vi "SetBTI.vi"(8 "error in (no error)":errorcluster, 10 "bti_mode":u8) -> (0 "error out":errorcluster)   [LabVIEW 2015, in "ESLSCDLL.lvlib"]
uses:
  ESLSCDLL.lvlib
  Globals.vi
  ESLSCDLL.dll
panel:
  # "Chooses trigger input for general trigger input (GTI)\t\n- 0: I\n\t- 1: S1\n\t- 2: S2\n\t- 3: Timer"
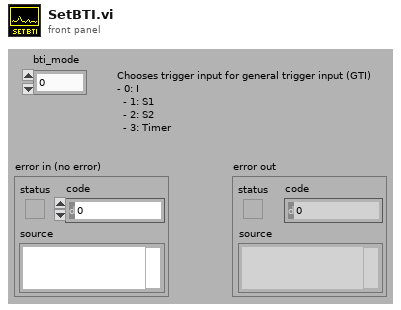
[diagram p1: front panel]
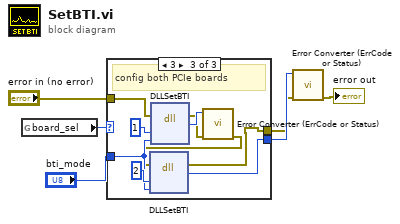
[diagram p0: block diagram]
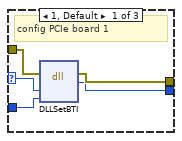
[diagram p2: hidden frame]
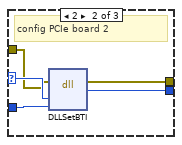
[diagram p3: hidden frame]
diagram:
  n1 = global read "Globals.vi" "board_sel"() -> (w1:u32)
  n2 = case shown="3" w1 {
    selector: w1 -> [w11 w16 _]
    tunnel: "bti_mode" -> [w10 w15 w23]
    tunnel: "error in (no error)" -> [w9 w14 w20]
    tunnel: [w7 w13 w17] -> w3
    tunnel: [w8 w12 w18] -> w2
    frame 1, Default {
      # "config PCIe board 1"
      n3 = dll-call lib="C:/Users/flori/Nextcloud/Dokumente/Stresing/Windows/lv64/board.vis/ESLSCDLL.dll" fn="DLLSetBTI" ("lwlscdll.dll:DLLRsTOREG")(error in=w9, "drv"=w11, "bti_mode"=w10) -> (error out=w8:errorcluster, "es_status_codes"=w7:i32)  [unwired: 4 in, 1 out]
    }
    frame 2 {
      # "config PCIe board 2"
      n4 = dll-call lib="C:/Users/flori/Nextcloud/Dokumente/Stresing/Windows/lv64/board.vis/ESLSCDLL.dll" fn="DLLSetBTI" ("lwlscdll.dll:DLLRsTOREG")(error in=w14, "drv"=w16, "bti_mode"=w15) -> (error out=w12:errorcluster, "es_status_codes"=w13:i32)  [unwired: 4 in, 1 out]
    }
    frame 3 {
      # "config both PCIe boards"
      n5 = dll-call lib="C:/Users/flori/Nextcloud/Dokumente/Stresing/Windows/lv64/board.vis/ESLSCDLL.dll" fn="DLLSetBTI" ("lwlscdll.dll:DLLRsTOREG")(error in=w20, "drv"=u32 1, "bti_mode"=w23) -> (error out=w21:errorcluster, "es_status_codes"=w22:i32)  [unwired: 4 in, 1 out]
      n6 = call "Error Converter (ErrCode or Status).vi"("error in (no error)"=w21, "error code"=w22) -> ("error out"=w19:errorcluster)  [unwired: 9 in]
      n7 = dll-call lib="C:/Users/flori/Nextcloud/Dokumente/Stresing/Windows/lv64/board.vis/ESLSCDLL.dll" fn="DLLSetBTI" ("lwlscdll.dll:DLLRsTOREG")(error in=w19, "drv"=u32 2, "bti_mode"=w23) -> (error out=w18:errorcluster, "es_status_codes"=w17:i32)  [unwired: 4 in, 1 out]
    }
  }
  n8 = call "Error Converter (ErrCode or Status).vi"("error in (no error)"=w2, "error code"=w3) -> ("error out"=→"error out":errorcluster)  [unwired: 9 in]
